vi "Get Subtype Description.vi"(8 "error in (no error)":errorcluster, 11 "String Assertion in":refnum<class "String Assertion.lvclass">) -> (0 "error out":errorcluster, 2 "Subtype Description":string, 3 "String Assertion out":refnum<class "String Assertion.lvclass">)   [LabVIEW 2020, in "MacroAssert.lvlib" / "String Assertion.lvclass"]
doc: "Gets the subtype description for <B>Step in</B>, which describes what the step's subtype does specifically."
uses:
  String Assertion.lvclass
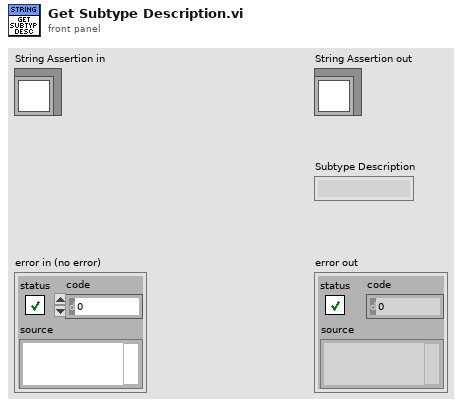
[diagram p1: front panel]
types:
  T1 = typedef "MacroAssert.lvlib/String Assertion.lvclass/String Assertion Type.ctl" = enum16{"String Ctl Value", "Ctl Caption Property", "Ctl Tip Strip Property", "Frontmost VI Name", "Frontmost Window Name"}
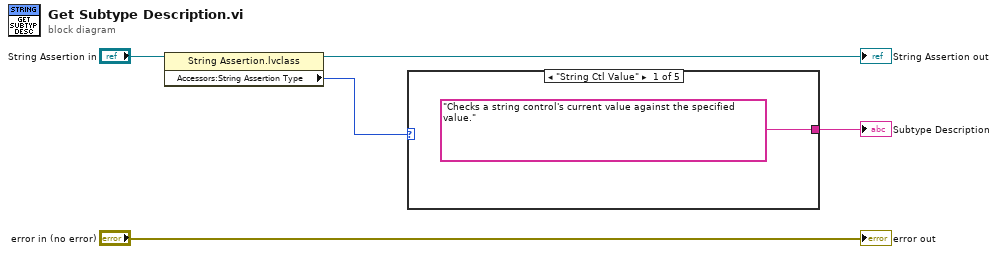
[diagram p0: block diagram]
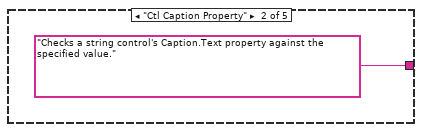
[diagram p2: hidden frame]
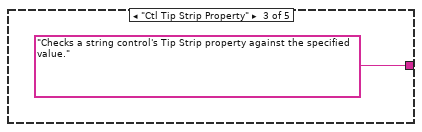
[diagram p3: hidden frame]
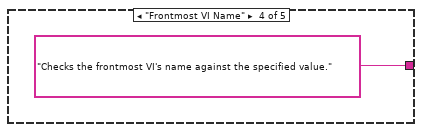
[diagram p4: hidden frame]
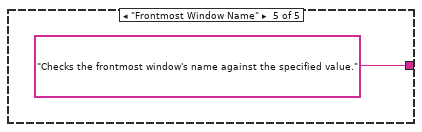
[diagram p5: hidden frame]
diagram:
  n1 = property class="String Assertion.lvclass"(reference="String Assertion in") -> (reference out=→"String Assertion out":refnum<class "String Assertion.lvclass">, "Accessors:String Assertion Type"=w5:T1)  [unwired: 1 in, 1 out]
  n2 = case shown="\"String Ctl Value\"" w5 {
    tunnel: ["Checks a string control's current value against the specified value." "Checks a string control's Caption.Text property against the specified value." "Checks a string control's Tip Strip property against the specified value." "Checks the frontmost VI's name against the specified value." "Checks the frontmost window's name against the specified value."] -> w1
    frame "String Ctl Value" {
    }
    frame "Ctl Caption Property" {
    }
    frame "Ctl Tip Strip Property" {
    }
    frame "Frontmost VI Name" {
    }
    frame "Frontmost Window Name" {
    }
  }
  "Subtype Description" <- w1
  "error out" <- "error in (no error)"
